vi "Keyence.Main-Scan.vi"(6 "get img (F)":bool, 7 "Idx":i32, 8 "error in":errorcluster, 9 "imgpath":path, 10 "Bank":u8, 11 "Retries (-1: Default)":i32=-1) -> (0 "error out":errorcluster, 2 "Code":T3, 3 "Final status":T1={"State"=enum."Init", "Ref"=refnum, "Bank"=0, "Version"="", "Model"="", "EndTS"=timestamp(0 s since 1904-01-01), "ImgPath"=path "", "Tuned"=FALSE})   [LabVIEW 2016]
uses:
  LowLevel/Keyence.CodeDetails.ctl
  Keyence.Data.Status.ctl
  Keyence.Data.Status.State.ctl
  Keyence.Action.ctl
  tools/EventLog/EventLog.EventSource.ctl
  tools/Translator/Translator.Message.ctl
  tools/EventLog/EventLog.CreateError(array).vi
  tools/Translator/Translator.Translate.Status (NoError).vi
  tools/Translator/Translator.FormatMessage.vi
  tools/EventLog/EventLog.New(array).vi
  tools/Translator/Translator.Global.vi
  tools/ErrorHandling/ErrorHandling.Create.vi
  LowLevel/Keyence.Global.vi
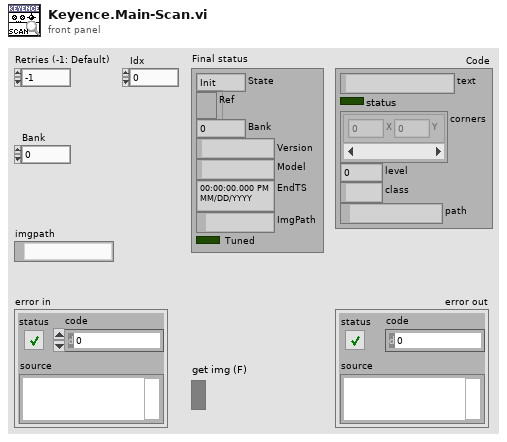
[diagram p1: front panel]
types:
  T1 = typedef "Keyence.Data.Status.ctl" = cluster{"State":T2, "Ref":refnum<k5>, "Bank":u8, "Version":string, "Model":string, "EndTS":timestamp, "ImgPath":path, "Tuned":bool}
  T2 = typedef "Keyence.Data.Status.State.ctl" = enum16{"First", "Init", "Reset", "Idle", "Scan", "Tune"}
  T3 = typedef "Keyence.CodeDetails.ctl" = cluster{"text":string, "status":bool, "corners":cluster{"X":i32, "Y":i32}[], "level":u8, "class":string, "path":path}
  T4 = typedef "Keyence.Action.ctl" = enum32{"idle", "constructor", "destructor", "--- Keyence ---", "Init", "Scan", "Tune"}
  T5 = typedef "Translator.Message.ctl" = enum16{"-", "Event confirmed", "Log out", "Log in", "Shutdown", "Cancel", "Start", "Begin time", "End time", "Duration", "Service Mode", "Ignore Results", "Serial Format", "On", "Off", "OK", "NOK", "NOK %s", "Home", "Work", "Close", "Open", "In progress...", "Missing", "Empty", "Hardware failure", "Initial", "Default", "Total", "Out of range", "Free disk space is below 1GB - contact technician", "Error %d >> %s", "Error %d >> %s >> %s", "Msg %d >> %s", "Laser msg %d %s", "Laser cmd error %s %d", "Laser cmd failed %s", "Laser cmd warning %s", "Laser disconnected", "Laser status %s", "Laser already started", "Laser job unkonwn %s", "Laser job missing %s", "Laser job select failure %s", "Unable to start laser printing (%s)", "Unable to stop laser printing (%s)", "Laser marking aborted", "Laser marking timeout", "Unable to reset Laser Interlock (%s)", "Unable to trigger Laser. Laser not ready (%s)", "Laser job '%s' coordinates not configured", "Starting %s", "Quitting %s", "Configured", "Initializing", "Quitting", "Loading", "Loaded %d results", "Loaded %d events", "Running", "Stopped", "Summary", "Laser", "Do you want to continue?", "Do you want to delete the configuration?", "The configuration is being used by an order. Unable to delete!", "Press confirm button", "Station is not based. Do you want to exit?", "Station requires changeover. Do you want to run the test?", "Test options are not set as default. Do you want to continue?", "Product not detected. Do you want to continue?", "Product scan failed. Do you want to continue?", "Calibration", "Log out?", "System", "All", "IDLE", "Translating...%s", "Not found", "Alarm %s", "Run", "Skip", "Abort", "Repeat", "Please wait...", "Database disconnected", "Database disconnected - changeover disabled!", "Login to database successful", "Login to database failed: %d; %s", "Unable to check the product status of reference %d - database disconnected", "Unable to set the product status of reference %d - database disconnected", "Variant file backup %s", "Read variant (%s)", "Result", "Station armed!", "Station requires changeover!", "Select reference number...", "EMERGENCY BUTTON - press Control button", "EMERGENCY DOOR - press Control button", "Resetting Emergency...", "Unable to reset safety circuit - Emergency Button pressed", "Unable to reset safety circuit - Emergency Side Door open", "Station not based", "Station based", "Station not empty", "Station basing...", "No order", "Press Start to begin new order", "Scanning new order", "Order NOK. Correct or scan again", "Order OK. Press Accept", "Order ready", "Revolver incorrect", "Fork incorrect", "Revolver missing", "Revolver empty", "Container missing", "Offline results", "Offline statistics", "Updating statistics %.1f %%", "DMC Configurator", "Door open", "Close the front door", "Press start button", "Done. Open the front door", "Running...", "Running...%.1f %%", "Pause %s", "Pause %s. NOK container missing", "Pause %s. OK container missing", "Pause %s. Revolver empty", "Pause %s. Revolver missing", "Pause %s. Revolver incorrect", "Pause %s. Fork missing", "Pause %s. Fork incorrect", "Pause %s. Too many failures", "Pause %s. One slot is not working", "Pause %s. Part order is done. Empty OK container", "Pause %s. Unable to move product to slot", "Pause %s. Unable to move back product pusher", "Pause %s. Unable to lift product", "Pause %s. Unable to move back product lifter", "Pause %s. Unable to move product arm to Work", "Pause %s. Unable to move product arm to NOK", "Pause %s. Unable to move product arm to OK", "Pause %s. Unable to unsuck the NOK product", "Pause %s. Unable to drop the NOK product", "Pause %s. Product OK missing", "Pause %s. Unable to unsuck the OK product", "Pause %s. Unable to drop the OK product", "Stopping...", "File '%s' is missing", "File '%s' is broken", "File '%s' is running", "Log file started (%s)", "Log file ended (%s)", "Log file stopped (%s)", "Log file ignored (%s)", "Log file exported (%s)", "Log file export failed (%s)", "Wrong serial number in log file", "Wrong reference number in log file", "Test steps are missing", "%s = %.3f", "Process param '%s' not found in DB", "Process param '%s' wrong order", "Process param '%s' value %.3f out of limits (%.3f; %.3f)", "Step%d param '%s' not found in DB", "Step%d param '%s' wrong order", "Step%d param '%s' value %.3f out of limits (%.3f; %.3f)", "Step%d EV '%s' not found in DB", "Step%d EV '%s' wrong order", "\"%s\" not found in DB", "\"%s\" wrong order", "\"%s\" value %.3f out of limits (%.3f; %.3f)", "\"%s\" not found in software", "Process init (%s)", "Process started", "Process restarted", "Process run", "Process done", "Process aborted", "Process aborted at work", "Process aborted at home", "Process error", "Process error at home", "Process error at work", "Process close", "Select plate from the order to process", "Do you want to start the process?", "Do you want to continue the process?", "There is unfinished order. Do you want to put the new order?", "Product %s %d OK", "Product %s %d NOK", "Unable to unload the slot %s. Product missing in the slot", "Unable to unload the slot %s. Product already in the arm", "Unable to accept the product as OK. Product missing in slot %s", "Unable to accept the product as OK. Product could not drop into the container at slot %s", "Unable to accept the product as NOK. Product could not drop into the container at slot %s", "Scan failed. Error %s", "Scan failed. Scanner disconnected", "Scan failed. Wrong Wabco number %d, limit (%d,%d)", "Scan failed. Wrong serial number %d, limit (%d,%d)", "Scan failed. Wrong date %d, limit (%d,%d)", "Scan failed. Wrong product wabco number %d (expected %d)", "Scan failed. Wrong product serial number %d (expected > 0)", "Scan OK %s", "Scan failed. Unable to determine table position (%s)", "Scan failed. Timeout", "Tune failed. Scanner disconnected", "Tune failed. Timeout", "%s = %d", "%s = %d->%d", "Unable to set %s = %.2f - Air Pressure Inside off", "Unable to set digital output '%s' = %d", "Unable to activate air pressure inside - timeout", "Unable to activate air pressure inside - aborted", "Unable to switch on Air Main Valve - Air Pressure Inlet off", "Unable to switch on Air Main Valve - Door open", "Unable to switch off Air Main Valve - timeout", "Unable to switch off Air Main Valve - aborted", "Unable to rotate Table - timeout", "Unable to rotate Table - aborted", "Unable to rotate Table - Product Move not in Home position", "Unable to rotate Table - Air Pressure Inside off", "Unable to rotate Table - Product Lift A not in Home position", "Unable to rotate Table - Product Lift B not in Home position", "Unable to rotate Table - unlock before movement timeout", "Unable to rotate Table - lock after movement timeout", "Unable to move Table Lock to %s position - timeout", "Unable to move Table Lock to %s position - aborted", "Unable to move Table Lock to %s position - Air Pressure Inside off", "Unable to move Table Lock to %s position - Table not in position", "Unable to move Product Lift A to %s position - timeout", "Unable to move Product Lift B to %s position - timeout", "Unable to move Product Lift A to %s position - aborted", "Unable to move Product Lift B to %s position - aborted", "Unable to move Product Lift A to %s position - Air Pressure Inside off", "Unable to move Product Lift B to %s position - Air Pressure Inside off", "Unable to move Product Lift A to %s position - Table not locked", "Unable to move Product Lift B to %s position - Table not locked", "Unable to move Product Lift A to %s position - Product Arm not in Work position", "Unable to move Product Lift B to %s position - Product Arm not in Work position", "Unable to set Product Suction Gripper %s to %s - timeout", "Unable to set Product Suction Gripper %s to %s - aborted", "Unable to set Product Suction Gripper %s to %s - Air Pressure Inside off", "Unable to set Product Suction Gripper %s to %s - Table slot unkown", "Unable to move Product Arm to %s position - timeout", "Unable to move Product Arm to %s position - aborted", "Unable to move Product Arm to %s position - Air Pressure Inside off", "Unable to move Product Arm to %s position - Product Lift A not in Home position", "Unable to move Product Arm to %s position - Product Lift B not in Home position", "Unable to move Product to %s position - timeout", "Unable to move Product to %s position - aborted", "Unable to move Product to %s position - Air Pressure Inside off", "Unable to move Product to %s position - Table not in position"}
  T6 = typedef "EventLog.EventSource.ctl" = enum16{"All", "Gui", "Ref", "File", "Arch", "Seq", "CPX", "DB", "Laser", "Scan.P", "Scan.O"}
  T7 = cluster{u8, "imgpath":path, "Retries (-1: Default)":i32, "get img (F)":bool}
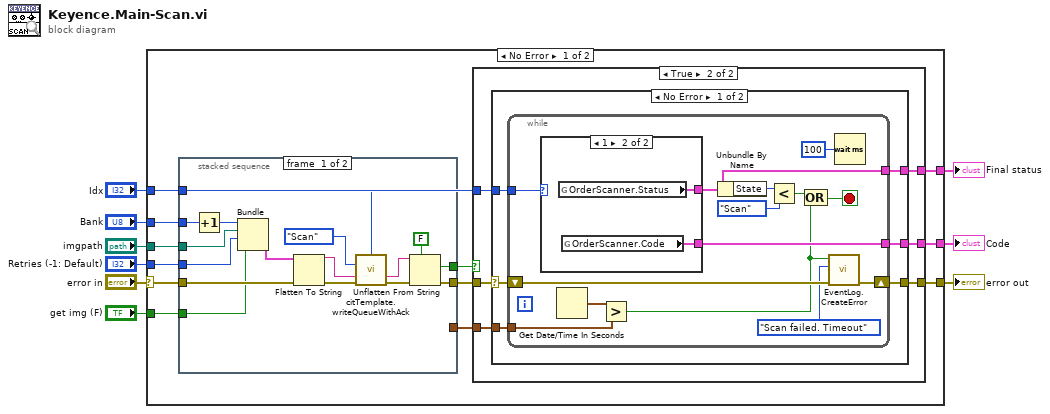
[diagram p0: block diagram]
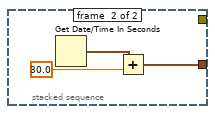
[diagram p2: hidden frame]
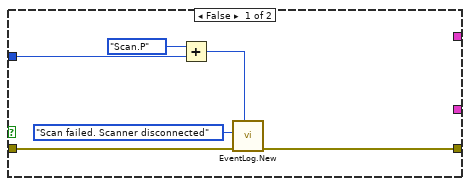
[diagram p3: hidden frame]
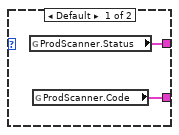
[diagram p4: hidden frame]
diagram:
  n1 = case shown="No Error" "error in" {
    selector: "error in" -> [w21 w78]
    tunnel: [w20 w78] -> w8
    tunnel: "Bank" -> [w16 _]
    tunnel: [w19 _] -> w6
    tunnel: "Idx" -> [w15 _]
    tunnel: "imgpath" -> [w13 _]
    tunnel: [w12 _] -> w3
    tunnel: "Retries (-1: Default)" -> [w11 _]
    tunnel: "get img (F)" -> [w10 _]
    frame No Error {
      n2 = stacked-sequence {
        tunnel: w21 -> [w37 _]
        tunnel: w15 -> [w33 _]
        tunnel: [w29 _] -> w18
        tunnel: [w28 _] -> w17
        tunnel: w16 -> [w27 _]
        tunnel: [_ w38] -> w14
        tunnel: w13 -> [w24 _]
        tunnel: w11 -> [w23 _]
        tunnel: w10 -> [w22 _]
        frame #0 {
          n3 = Increment(x=w27) -> (x+1=w26:u8)
          n4 = Bundle(w26, "imgpath"=w24, "Retries (-1: Default)"=w23, "get img (F)"=w22) -> (w25:T7)  [unwired: 1 in]
          n5 = Flatten To String(anything=w25, error in (no error)=w37) -> (data string=w35:string, error out=w36:errorcluster)  [unwired: 2 in, 1 out]
          n6 = call "citTemplate.writeQueueWithAck.vi"("instance (0)"=w33, "event in"=Keyence.Action."Scan" ("Action"), "(flatten) data in"=w35, "error in (no error)"=w36) -> ("notification data"=w31:string, "error out"=w32:errorcluster)  [unwired: 9 in, 1 out]
          n7 = Unflatten From String(type=FALSE, binary string=w31, error in (no error)=w32) -> (value=w28:bool, error out=w29:errorcluster)  [unwired: 2 in, 1 out]
        }
        frame #1 {
          n8 = Get Date/Time In Seconds() -> (seconds since 1Jan1904=w40:timestamp)
          n9 = Add(x=w40, y=30.0) -> (x+y=w38:timestamp)
        }
      }
      n10 = case shown="True" w17 {
        tunnel: w18 -> [w45 w52]
        tunnel: [w44 w51] -> w20
        tunnel: [_ w50] -> w19
        tunnel: w15 -> [w43 w49]
        tunnel: w14 -> [_ w48]
        tunnel: [_ w47] -> w12
        frame False {
          n11 = Add(x=EventLog.EventSource."Scan.P" ("Source (All)"), y=w43) -> (x+y=w41:i32)
          n12 = call-poly "EventLog.New.vi"("Source (All)"=w41, "error in (no error)"=w45, "Message (-)"=Translator.Message."Scan failed. Scanner disconnected") -> ("error out"=w44:errorcluster)  [unwired: 7 in, 1 out]
        }
        frame True {
          n13 = case shown="No Error" w52 {
            selector: w52 -> [w57 w77]
            tunnel: [w56 w77] -> w51
            tunnel: [w58 _] -> w50
            tunnel: w49 -> [w55 _]
            tunnel: w48 -> [w54 _]
            tunnel: [w53 _] -> w47
            frame No Error {
              n14 = while {
                tunnel: [w68] -> w58
                shift-right: [w62] -> w56
                shift-left: w57 -> [w67]
                tunnel: w55 -> [w66]
                tunnel: w54 -> [w65]
                tunnel: [w59] -> w53
                stop <- w63 stop-if-true
                n15 = case shown="1" w66 {
                  tunnel: [w74 w76] -> w59
                  tunnel: [w73 w75] -> w68
                  frame Default {
                    n16 = global read "Keyence.Global.vi" "ProdScanner.Status"() -> (w74:T1)
                    n17 = global read "Keyence.Global.vi" "ProdScanner.Code"() -> (w73:T3)
                  }
                  frame 1 {
                    n18 = global read "Keyence.Global.vi" "OrderScanner.Status"() -> (w76:T1)
                    n19 = global read "Keyence.Global.vi" "OrderScanner.Code"() -> (w75:T3)
                  }
                }
                n20 = Get Date/Time In Seconds() -> (seconds since 1Jan1904=w64:timestamp)
                n21 = Greater?(x=w64, y=w65) -> (0:w61:bool)
                n22 = Unbundle By Name(w59) -> ("State"=w72:T2)
                n23 = Less?(x=w72, y=Keyence.Data.Status.State."Scan") -> (x < y?=w70:bool)
                n24 = Compound Arithmetic op=OR(w70, w61) -> (w63:bool)
                n25 = call-poly "EventLog.CreateError.vi"("error in"=w67, "msg"=Translator.Message."Scan failed. Timeout", "create (T)"=w61) -> ("error out"=w62:errorcluster)  [unwired: 7 in, 1 out]
                n26 = Wait (ms)(milliseconds to wait=u32 100) -> ()  [unwired: 1 out]
              }
            }
            frame Error {
            }
          }
        }
      }
    }
    frame Error {
    }
  }
  "error out" <- w8
  "Code" <- w6
  "Final status" <- w3
